vi "test.vi"(8 "error in (no error)":errorcluster) -> (0 "error out":errorcluster, 3 "Full Report":string)   [LabVIEW 2018, in "labview_json_tests.lvlib"]
uses:
  labview_json_tests.lvlib
panel:
  out "ms Avg Dump":dbl
  out "ms Avg Load":dbl
  in  "Show Passed? (F)":bool
  out "All Passed?":bool
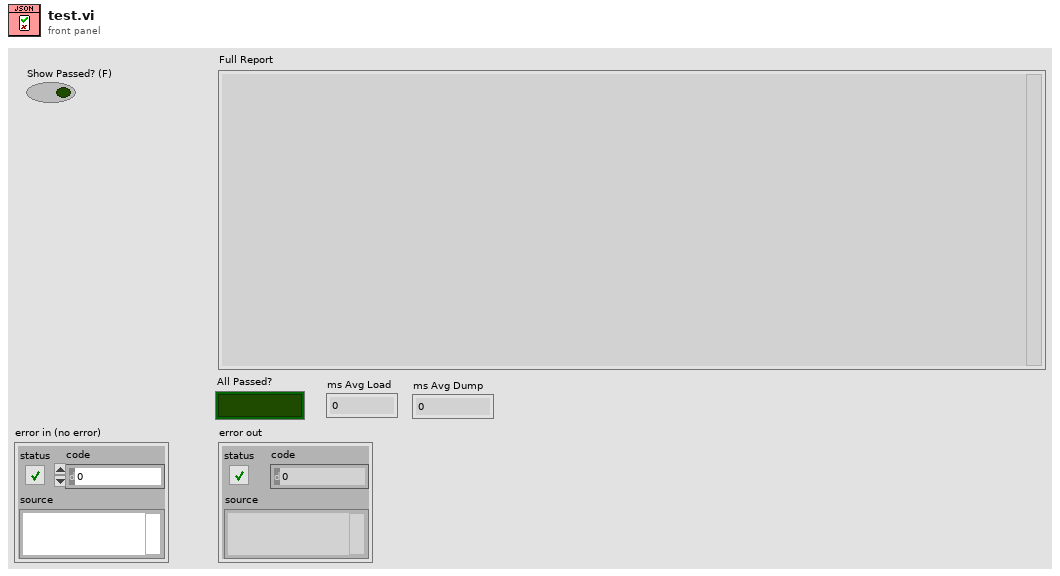
[diagram p1: front panel]
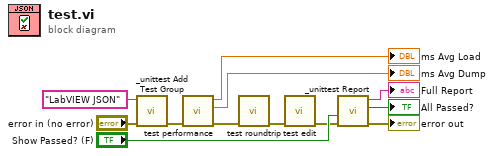
[diagram p0: block diagram]
diagram:
  n1 = call "_unittest Add Test Group.vi"("error in (no error)"="error in (no error)", "Test Group"="LabVIEW JSON" ("Test Case")) -> ("error out"=w6:errorcluster)  [unwired: 9 in]
  n2 = call "test performance.vi"("error in (no error)"=w6) -> ("error out"=w3:errorcluster, "ms Avg Dump"=→"ms Avg Dump":dbl, "ms Avg Load"=→"ms Avg Load":dbl)  [unwired: 8 in]
  n3 = call "test roundtrip.vi"("error in (no error)"=w3) -> ("error out"=w2:errorcluster)  [unwired: 9 in, 1 out]
  n4 = call "test edit.vi"("error in (no error)"=w2) -> ("error out"=w1:errorcluster)  [unwired: 9 in, 1 out]
  n5 = call "_unittest Report.vi"("error in (no error)"=w1, "Show Passed? (F)"="Show Passed? (F)") -> ("error out"=→"error out":errorcluster, "All Passed?"=→"All Passed?":bool, "Full Report"=→"Full Report":string)  [unwired: 7 in]
